vi "Read configuration.vi"(8 "error in":errorcluster, 11 "E2E Tag Exchange editor node in":refnum<class "E2E Tag Exchange editor node.lvclass">) -> (0 "error out":errorcluster, 2 "configuration":refnum<class "NISE_CEF_serializable configuration.lvclass">, 3 "E2E Tag Exchange editor node out":refnum<class "E2E Tag Exchange editor node.lvclass">)   [LabVIEW 2015, in "E2E Tag Exchange editor node.lvclass"]
uses:
  E2E Tag Exchange editor node.lvclass
  <vilib>/NI/Configuration Framework/serializable configuration/NISE_CEF_serializable configuration.lvclass
  E2E Tag Exchange editor node.lvclass/E2E Tag Exchange editor node.ctl
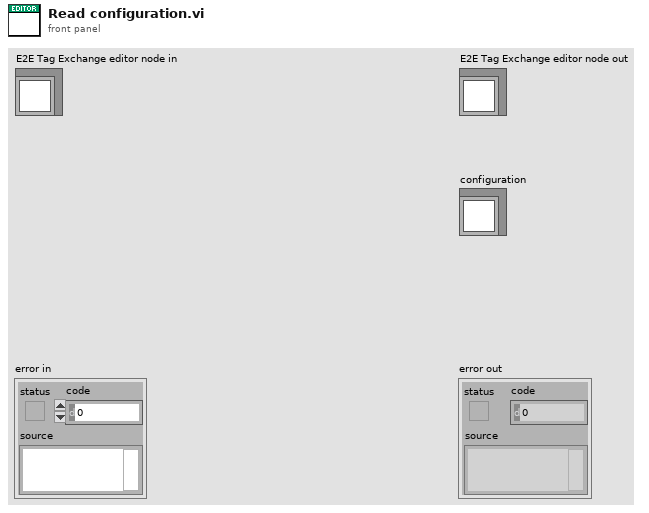
[diagram p1: front panel]
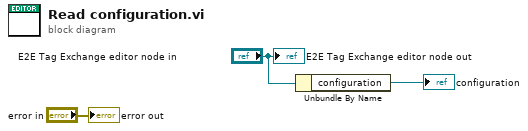
[diagram p0: block diagram]
diagram:
  n1 = Unbundle By Name("E2E Tag Exchange editor node in") -> ("configuration"=→"configuration":refnum<class "E2E Tag Exchange configuration.lvclass">)
  "error out" <- "error in"
  "E2E Tag Exchange editor node out" <- "E2E Tag Exchange editor node in"
